vi "RSZVB Get UI Port Next State.vi"(8 "error in (no error)":errorcluster {"code" format="%.0x"}, 9 "Port (1)":i32=1, 11 "VISA session":refnum<visa-resource-name>) -> (0 "error out":errorcluster {"code" format="%.0x"}, 2 "Next State":i32, 3 "dup VISA session":refnum<visa-resource-name>)   [LabVIEW 2011]
doc: "Returns the state of the output ports (pin 3 or 4) of the Universal Interface connector after the next negative pulse on the Input 1 line (pin 2). \n\nRemote-control command(s):\nCONTrol:HANDler:OUTPut<port>:USER?"
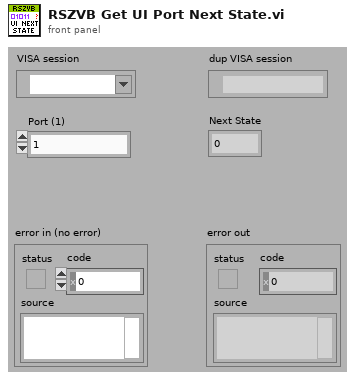
[diagram p1: front panel]
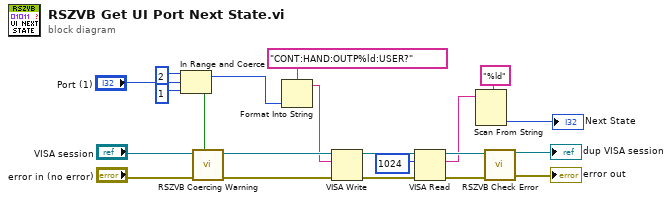
[diagram p0: block diagram]
diagram:
  n1 = In Range and Coerce(upper limit=2, x="Port (1)", lower limit=1) -> (coerced(x)=w7:i32, In Range?=w10:bool)
  n2 = call "RSZVB Coercing Warning.vi"("In Range?"=w10, "error in (no error)"="error in (no error)", "VISA session"="VISA session") -> ("error out"=w13:errorcluster, "dup VISA session"=w12:refnum<visa-resource-name>)  [unwired: 7 in]
  n3 = Format Into String(format string="CONT:HAND:OUTP%ld:USER?", w7) -> (resulting string=w11:string)  [unwired: 2 in, 1 out]
  n4 = VISA Write(VISA resource name=w12, write buffer=w11, error in (no error)=w13) -> (VISA resource name out=w19:refnum<visa-resource-name>, error out=w21:errorcluster)  [unwired: 1 out]
  n5 = VISA Read(VISA resource name=w19, byte count=u32 1024 ("byte count (0)"), error in (no error)=w21) -> (VISA resource name out=w18:refnum<visa-resource-name>, read buffer=w8:string, error out=w17:errorcluster)  [unwired: 1 out]
  n6 = Scan From String(format string="%ld", input string=w8) -> (output 1=→"Next State":i32)  [unwired: 3 in, 3 out]
  n7 = call "RSZVB Check Error.vi"("error in (no error)"=w17, "VISA session"=w18) -> ("error out"=→"error out":errorcluster, "dup VISA session"=→"dup VISA session":refnum<visa-resource-name>)  [unwired: 8 in]
